vi "Window-Larger image.vi"(9 "Image name":string="Vid 1", 10 "Open maximised":bool) -> ()   [LabVIEW 2017]
uses:
  User Interface/Visualisation/Timelapse Viewer/Globals/gl_Time series viewer globals.vi
panel:
  out "Rel time (ms)":u32 format="Relative time: %.0f ms"
  out "Vid":T1(plugin-control)
  out "Stop":bool
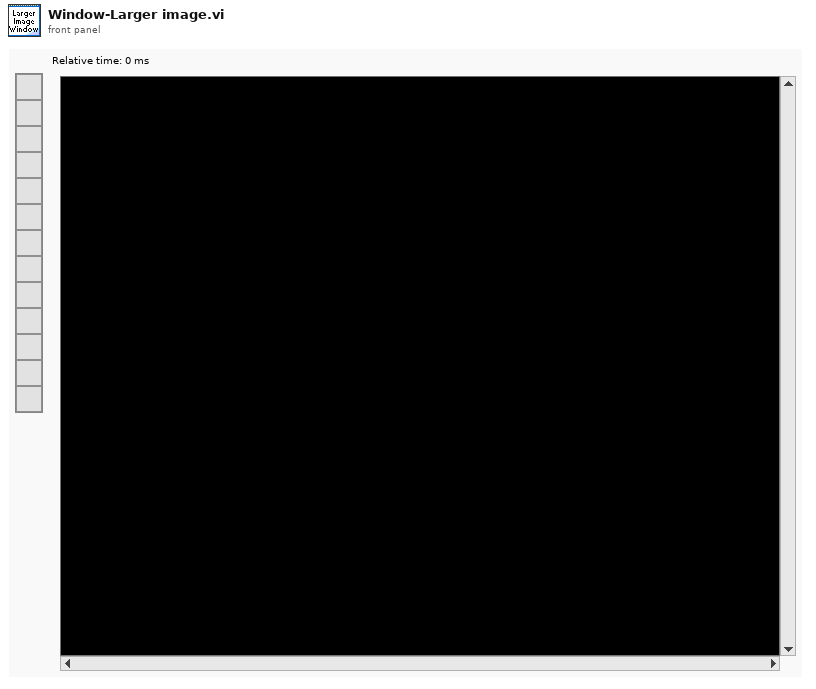
[diagram p1: front panel]
types:
  T1 = typedef "IMAQ Image.ctl" = refnum<image>
  T2 = enum16{"None", "Release queue", "Obtain queue", "Enqueue", "Get status", "Set status"}
  T3 = enum32{"Invalid", "Standard", "Closed", "Hidden", "Minimized", "Maximized"}
  T4 = typedef "Larger windows queues interface cluster.ctl" = cluster{"error out 1":errorcluster, "Window 1 is open":bool, "error out 2":errorcluster, "Window 2 is open":bool, "error out 3":errorcluster, "Window 3 is open":bool, "error out 4":errorcluster, "Window 4 is open":bool, "Larger image window queue 1":T5, "Larger image window queue 2":T5, "Larger image window queue 3":T5, "Larger image window queue 4":T5}
  T5 = typedef "Larger window queue ref.ctl" = refnum<queue>
  T6 = typedef "Larger window queue cluster.ctl" = cluster{"Vid":T1, "Rel time (ms)":u32}
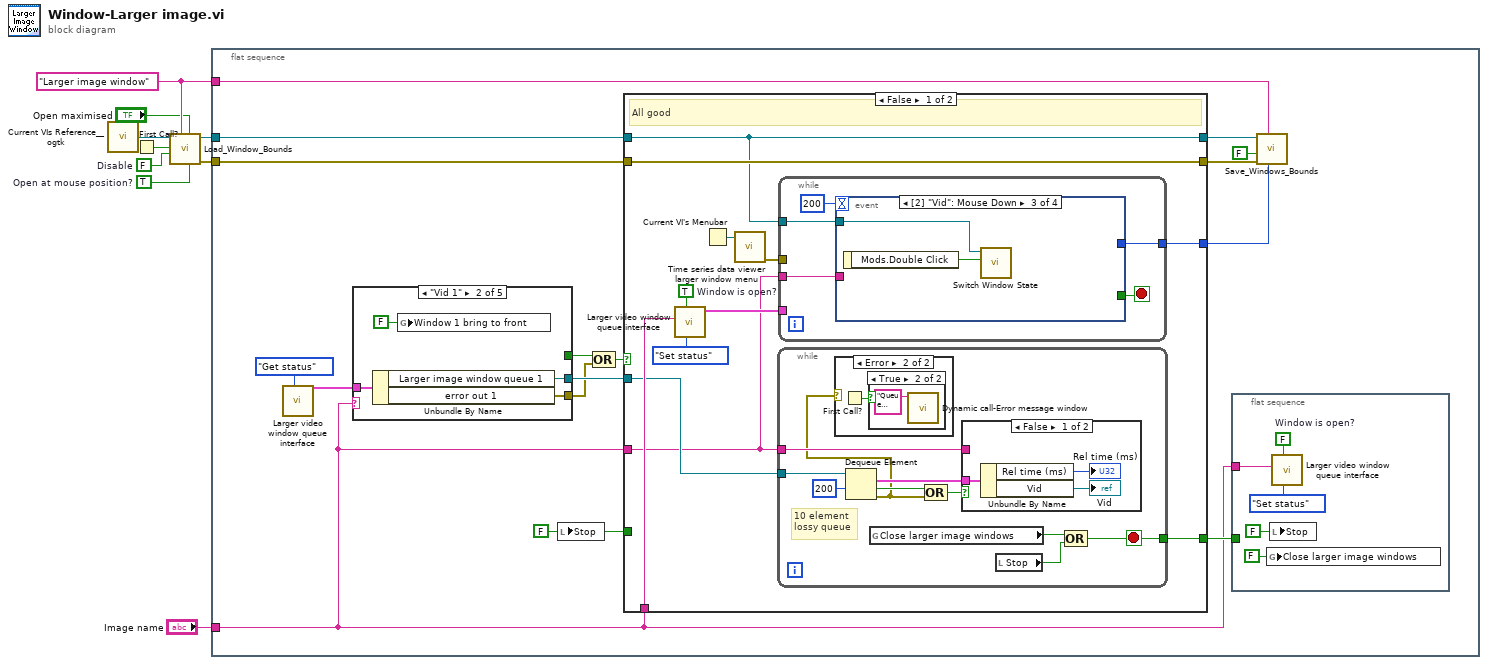
[diagram p0: block diagram]
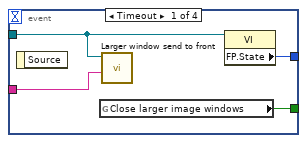
[diagram p2: hidden frame]
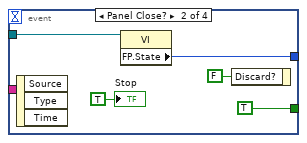
[diagram p3: hidden frame]
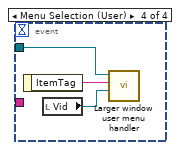
[diagram p4: hidden frame]
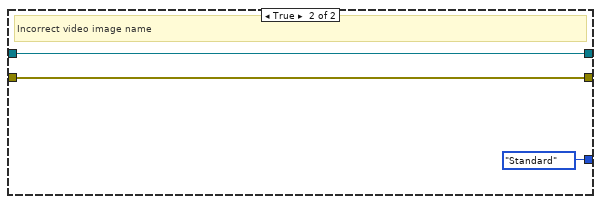
[diagram p8: hidden frame]
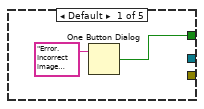
[diagram p9: hidden frame]
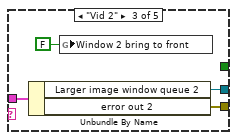
[diagram p10: hidden frame]
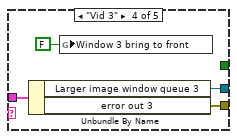
[diagram p11: hidden frame]
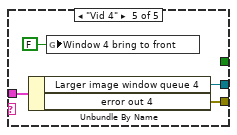
[diagram p12: hidden frame]
diagram:
  w3 = TRUE  # Open at mouse position?
  w7 = FALSE  # Disable
  w5 = "Larger image window" ("Window Name (i.e. Key)")
  n1 = call <userlib>:"Current VIs Reference__ogtk.vi"() -> ("Current VI's reference"=w9:refnum<vi>)  [unwired: 5 in]
  n2 = First Call?() -> (First Call?: T/F=w8:bool)
  n3 = call "Load_Window_Bounds.vi"("Open at mouse position?"=w3, "Open maximised?"="Open maximised", "Window Name (i.e. Key)"=w5, "Disable"=w7, "First Call"=w8, "Window VI's Ref"=w9) -> ("error out"=w6:errorcluster, "reference out"=w4:refnum<vi>)  [unwired: 2 in, 2 out]
  n4 = flat-sequence {
    tunnel: w6 -> [w21]
    tunnel: w5 -> [w19]
    tunnel: w4 -> [w11]
    tunnel: "Image name" -> [w15]
    frame #0 {
      w17 = FALSE ("Stop")
      n5 = call "Larger video window queue interface.vi"("Function"=T2."Get status") -> ("Output cluster"=w14:T4)  [unwired: 10 in]
      n6 = case shown="\"Vid 1\"" w15 {
        tunnel: [w80 _ _ _ _] -> w23
        tunnel: w14 -> [_ w85 w89 w93 w97]
        tunnel: [_ w84 w88 w92 w96] -> w13
        tunnel: [_ w83 w87 w91 w95] -> w12
        frame Default {
          n7 = One Button Dialog(message="Error. Incorrect image name.") -> (true=w80:bool)  [unwired: 1 in]
        }
        frame "Vid 1" {
          n8 = Unbundle By Name(w85) -> ("Larger image window queue 1"=w84:T5, "error out 1"=w83:errorcluster)
          n9 = global write "gl_Time series viewer globals.vi" "Window 1 bring to front"(FALSE ("Window 1 bring to front")) -> ()
        }
        frame "Vid 2" {
          n10 = Unbundle By Name(w89) -> ("Larger image window queue 2"=w88:T5, "error out 2"=w87:errorcluster)
          n11 = global write "gl_Time series viewer globals.vi" "Window 2 bring to front"(FALSE ("Window 1 bring to front")) -> ()
        }
        frame "Vid 3" {
          n12 = Unbundle By Name(w93) -> ("Larger image window queue 3"=w92:T5, "error out 3"=w91:errorcluster)
          n13 = global write "gl_Time series viewer globals.vi" "Window 3 bring to front"(FALSE ("Window 1 bring to front")) -> ()
        }
        frame "Vid 4" {
          n14 = Unbundle By Name(w97) -> ("Larger image window queue 4"=w96:T5, "error out 4"=w95:errorcluster)
          n15 = global write "gl_Time series viewer globals.vi" "Window 4 bring to front"(FALSE ("Window 1 bring to front")) -> ()
        }
      }
      n16 = local write "Stop"(w17) -> ()
      n17 = Compound Arithmetic op=OR(w23, w12) -> (w22:bool)
      n18 = case shown="False" w22 {
        tunnel: w15 -> [w33 _]
        tunnel: [w42 _] -> w24
        tunnel: w21 -> [w41 w79]
        tunnel: [w41 w79] -> w20
        tunnel: w11 -> [w31 w78]
        tunnel: [w31 w78] -> w18
        tunnel: w17 -> [_ _]
        tunnel: w15 -> [w37 _]
        tunnel: w13 -> [w36 _]
        tunnel: [w32 T3."Standard" ("FP.State")] -> w10
        frame False {
          w40 = TRUE  # Window is open?
          # "All good"
          n19 = call "Larger video window queue interface.vi"("Function"=T2."Set status", "Window is open?"=w40, "Image name"=w37) -> ("Output cluster"=w38:T4)  [unwired: 8 in]
          n20 = Current VI's Menubar() -> (w35:refnum<k9>)
          n21 = call "Time series data viewer larger window menu.vi"("menu"=w35) -> ("error out"=w34:errorcluster)  [unwired: 9 in, 1 out]
          n22 = while {
            tunnel: w33 -> [w66]
            tunnel: [w69] -> w42
            tunnel: w36 -> [w65]
            stop <- w69 stop-if-true
            # "10 element\nlossy queue"
            n23 = Dequeue Element(queue=w65, timeout in ms (-1)=200) -> (element=w71:T6, timed out?=w64:bool, error out=w62:errorcluster)  [unwired: 1 in, 1 out]
            n24 = case shown="Error" w62 {
              frame No Error {
              }
              frame Error {
                n25 = First Call?() -> (First Call?: T/F=w72:bool)
                n26 = case shown="True" w72 {
                  frame False {
                  }
                  frame True {
                    n27 = call "Dynamic call-Error message window.vi"("Error Message"="Queue error in the pop up image window.") -> ()  [unwired: 10 in, 1 out]
                  }
                }
              }
            }
            n28 = global read "gl_Time series viewer globals.vi" "Close larger image windows"() -> (w68:bool)
            n29 = Compound Arithmetic op=OR(w64, w62) -> (w63:bool)
            n30 = case shown="False" w63 {
              tunnel: w71 -> [w76 _]
              tunnel: w66 -> [_ _]
              frame False {
                n31 = Unbundle By Name(w76) -> ("Rel time (ms)"=→"Rel time (ms)":u32, "Vid"=→"Vid":T1)
              }
              frame True {
              }
            }
            n32 = local read "Stop"() -> (w67:bool)
            n33 = Compound Arithmetic op=OR(w68, w67) -> (w69:bool)
          }
          n34 = while {
            tunnel: w38 -> [_]
            tunnel: w34 -> [_]
            tunnel: w31 -> [w45]
            tunnel: w33 -> [w44]
            tunnel: [w43] -> w32
            stop <- w47 stop-if-true
            n35 = event shown="[2] \"Vid\": Mouse Down" {
              selector: _ -> [_ _ _ _]
              dyn-events: _ -> [_ _ _ _]
              timeout: 200 -> [_ _ _ _]
              tunnel: [w51 TRUE ("Close larger image window") _ _] -> w47
              tunnel: w45 -> [w48 w53 w58 w59]
              tunnel: w44 -> [w50 _ _ _]
              tunnel: [w49 w54 _ _] -> w43
              event Timeout {
                n36 = event-data() -> ()  [unwired: 1 in, 1 out]
                n37 = global read "gl_Time series viewer globals.vi" "Close larger image windows"() -> (w51:bool)
                n38 = call "Larger window send to front.vi"("Image name"=w50, "Window VI's Ref"=w48) -> ()  [unwired: 10 in]
                n39 = property class="VI"(reference=w48) -> ("FP.State"=w49:T3)  [unwired: 1 in, 2 out]
              }
              event Panel Close? {
                n40 = event-data() -> ()  [unwired: 1 in, 3 out]
                n41 = property class="VI"(reference=w53) -> ("FP.State"=w54:T3)  [unwired: 1 in, 2 out]
                n42 = event-data("Discard?"=FALSE) -> ()  [unwired: 1 in, 1 out]
                "Stop" <- TRUE
              }
              event "Vid": Mouse Down {
                n43 = event-data() -> ("Mods.Double Click"=w57:bool)  [unwired: 1 in]
                n44 = call "Switch Window State.vi"("Enable (T)"=w57, "Window VI's Ref"=w58) -> ()  [unwired: 9 in, 1 out]
              }
              event Menu Selection (User) {
                n45 = event-data() -> ("ItemTag"=w60:string)  [unwired: 1 in]
                n46 = local read "Vid"() -> (w61:T1)
                n47 = call "Larger window user menu handler.vi"("Image"=w61, "ItemTag"=w60, "Window VI's Ref"=w59) -> ()  [unwired: 9 in]
              }
            }
          }
        }
        frame True {
          # "Incorrect video image name"
        }
      }
      n48 = flat-sequence {
        tunnel: w24 -> [_]
        tunnel: w15 -> [w26]
        frame #0 {
          w27 = FALSE  # Window is open?
          n49 = global write "gl_Time series viewer globals.vi" "Close larger image windows"(FALSE ("Close larger image window")) -> ()
          n50 = local write "Stop"(FALSE ("Stop")) -> ()
          n51 = call "Larger video window queue interface.vi"("Function"=T2."Set status", "Window is open?"=w27, "Image name"=w26) -> ()  [unwired: 8 in, 1 out]
        }
      }
      n52 = call "Save_Windows_Bounds.vi"("FP.State"=w10, "Window Name (i.e. Key)"=w19, "error in"=w20, "Front Panel Window:Open"=FALSE, "Window VI's Ref"=w18) -> ()  [unwired: 6 in, 1 out]
    }
  }
